vi "get_Frame_simple.vi"() -> ()   [LabVIEW 2012]
panel:
  out "statusFlags":u8
  out "x-y":u32
  in  "numOfFrame":u16
  out "Waveform Graph":u16[][](graph)
  in  "stop":bool
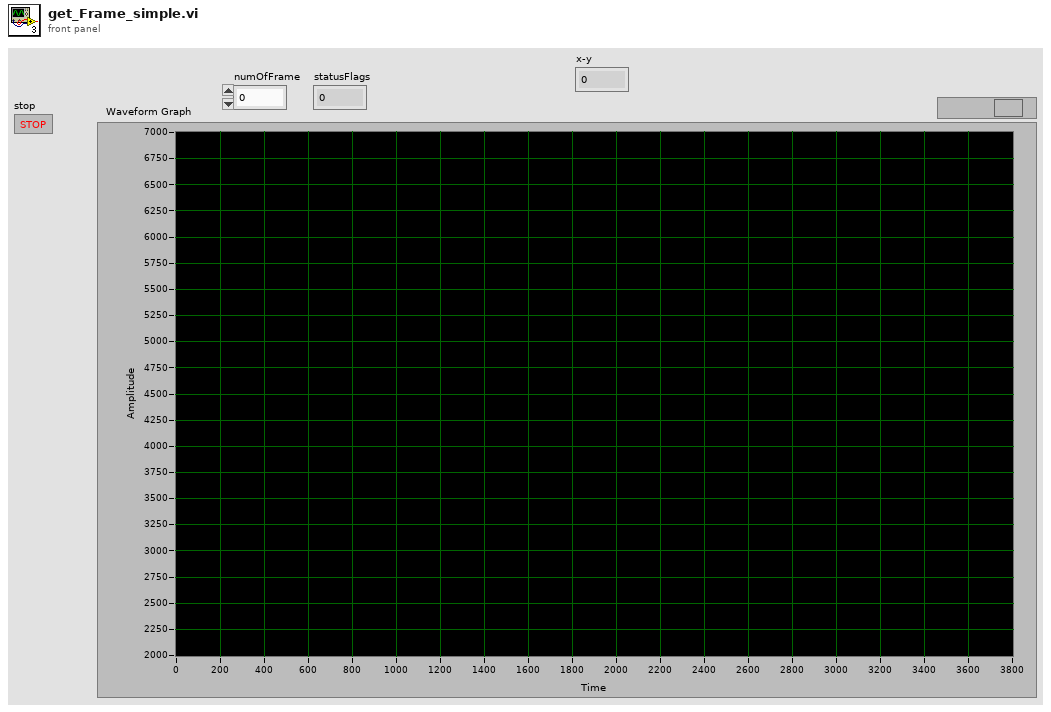
[diagram p1: front panel]
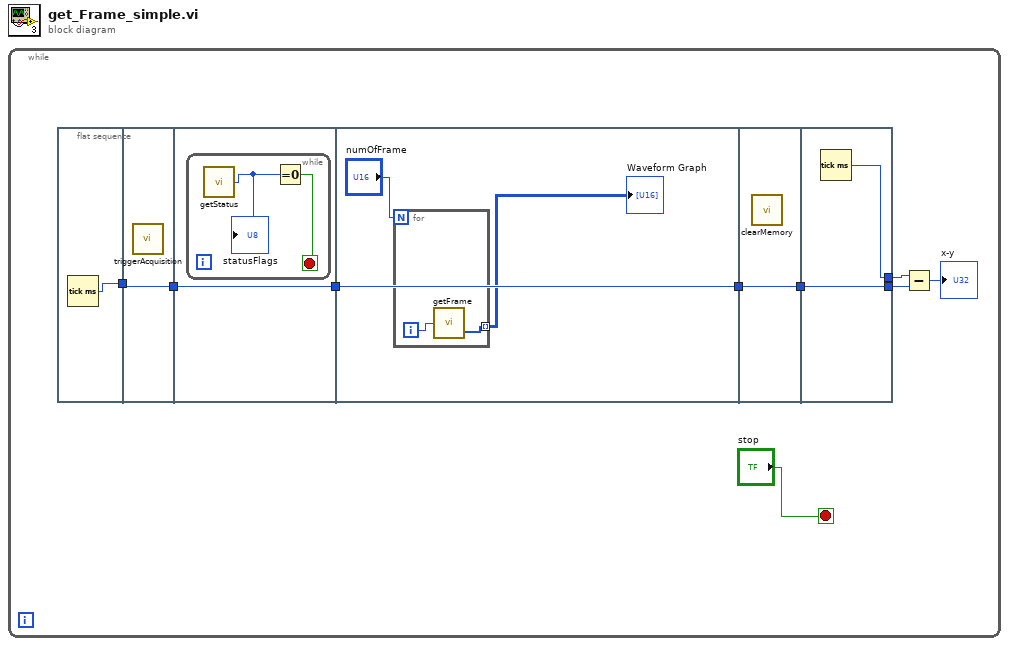
[diagram p0: block diagram]
diagram:
  n1 = while {
    stop <- "stop" stop-if-true
    n2 = flat-sequence {
      tunnel: [w10] -> w7
      tunnel: [w11] -> w6
      tunnel: w7 -> [w11]
      tunnel: w6 -> [w12]
      tunnel: [w12] -> w5
      tunnel: [w17] -> w8
      tunnel: w5 -> [w17]
      tunnel: [w20] -> w9
      tunnel: w8 -> [w20]
      tunnel: w9 -> [w22]
      tunnel: [w22] -> w3
      tunnel: [w21] -> w2
      frame #0 {
        n3 = Tick Count (ms)() -> (millisecond timer value=w10:u32)
      }
      frame #1 {
        n4 = call "triggerAcquisition.vi"() -> ()  [unwired: 1 out]
      }
      frame #2 {
        n5 = while {
          stop <- w14 stop-if-true
          n6 = call "getStatus.vi"() -> ("statusFlags"=w13:u8)  [unwired: 2 out]
          "statusFlags" <- w13
          n7 = Equal To 0?(x=w13) -> (x = 0?=w14:bool)
        }
      }
      frame #3 {
        n8 = for {
          N: "numOfFrame" -> [_]
          tunnel: [w19] -> w15 mode=indexing
          i -> [w18]
          n9 = call "getFrame.vi"("numOfFrame"=w18) -> ("framePixelsBuffer"=w19:u16[])  [unwired: 1 out]
        }
        "Waveform Graph" <- w15
      }
      frame #4 {
        n10 = call "clearMemory.vi"() -> ()  [unwired: 1 out]
      }
      frame #5 {
        n11 = Tick Count (ms)() -> (millisecond timer value=w21:u32)
      }
    }
    n12 = Subtract(x=w2, y=w3) -> (x-y=→"x-y":u32)
  }
